vi "Checksum Calculate.vi"(11 "Command in":string) -> (0 "Checksum (byte)":u8 format="%.0x", 1 "Checksum (string)":string, 2 "Command out (with checksum)":string, 3 "Command out (original)":string)   [LabVIEW 2017, in "Samwontech TEMP2xxx.lvlib"]
uses:
  <instrlib>/Samwontech TEMP2xxx/Samwontech TEMP2xxx.lvlib
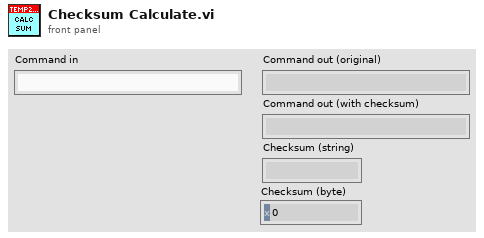
[diagram p1: front panel]
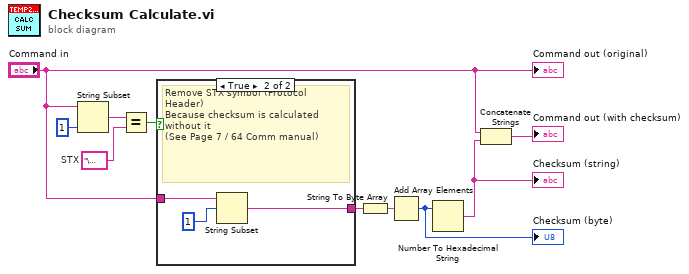
[diagram p0: block diagram]
diagram:
  w8 = "\u0002"  # STX
  n1 = String Subset(string="Command in", length (rest)=1 ("length (rest)")) -> (substring=w9:string)  [unwired: 1 in]
  n2 = Equal?(x=w9, y=w8) -> (x = y?=w7:bool)
  n3 = case shown="True" w7 {
    tunnel: "Command in" -> [w11 w14]
    tunnel: [w11 w12] -> w5
    frame False {
    }
    frame True {
      # "Remove STX symbol (Protocol Header)\nBecause checksum is calculated without it \n(See Page 7 / 64 Comm manual)"
      n4 = String Subset(string=w14, offset (0)=1) -> (substring=w12:string)  [unwired: 1 in]
    }
  }
  n5 = String To Byte Array(string=w5) -> (unsigned byte array=w6:u8[])
  n6 = Add Array Elements(numeric array=w6) -> (sum=w1:u8)
  "Checksum (byte)" <- w1
  n7 = Number To Hexadecimal String(2:w1) -> (0:w3:string)  [unwired: 1 in]
  "Checksum (string)" <- w3
  n8 = Concatenate Strings("Command in", w3) -> (→"Command out (with checksum)":string)
  "Command out (original)" <- "Command in"
